vi "S4GUI.vi"() -> ()   [LabVIEW 2018] (continued)
            n2911 = call-dynamic "Write Temperature.vi"("error in (no error)"=w7074, "Temperature"="Target Temp 4", "Interface in"=w7075) -> ("error out"=w7070:errorcluster, "Interface out"=w7073:refnum<class "Interface.lvclass">)  [unwired: 7 in]
            n2912 = call-dynamic "Write Interface.vi"("error in (no error)"=w7070, "Interface.lvclass"=w7073, "Channel in"=w7072) -> ("error out"=w7069:errorcluster, "Channel out"=w7071:refnum<class "Channel.lvclass">)  [unwired: 7 in]
            n2913 = call-dynamic "Read State Machine.vi"("error in (no error)"=w7069, "Device in"=w7071) -> ("error out"=w7092:errorcluster, "State Machine.lvclass"=w7093:refnum<class "State Machine.lvclass">, "Device out"=w7089:refnum<class "Channel.lvclass">)  [unwired: 7 in]
            n2914 = call "Next State.vi"("error in (no error)"=w7092, "New_State"=u32 35, "State Machine in"=w7093) -> ("error out"=w7087:errorcluster, "State Machine out"=w7090:refnum<class "State Machine.lvclass">)  [unwired: 7 in]
            n2915 = call-dynamic "Write State Machine.vi"("error in (no error)"=w7087, "State Machine.lvclass"=w7090, "Device in"=w7089) -> ("error out"=w7083:errorcluster, "Device out"=w7082:refnum<class "Channel.lvclass">)  [unwired: 7 in]
            n2916 = call-dynamic "Write Channel.vi"("error in (no error)"=w7083, "Channel.lvclass"=w7082, "Acquisition in"=w7088) -> ("error out"=w7084:errorcluster, "Acquisition out"=w7086:refnum<class "Acquisition.lvclass">)  [unwired: 7 in]
            n2917 = call-dynamic "Write AcquisitionD.vi"("error in (no error)"=w7084, "Acquisition.lvclass"=w7086, "S4ACS_GUI in"=w7085) -> ("error out"=w7079:errorcluster, "S4ACS_GUI out"=w7078:refnum<class "S4GUI.lvclass">)  [unwired: 7 in]
          }
        }
      }
      event "Avança Estado": Value Change {
        n2918 = event-data() -> ()  [unwired: 1 in, 4 out]
        n2919 = call-dynamic "Read Sync Box.lvclass.vi"("error in (no error)"=w7104, "SPARC4_AC in"=w7105) -> ("error out"=w7117:errorcluster, "Sync Box.lvclass"=w7118:refnum<class "Sync Box.lvclass">, "SPARC4_AC out"=w7109:refnum<class "S4GUI.lvclass">)  [unwired: 7 in]
        n2920 = call-dynamic "Read Trigger.lvclass.vi"("error in (no error)"=w7117, "Sync Box in"=w7118) -> ("error out"=w7115:errorcluster, "Trigger.lvclass"=w7116:refnum<class "Trigger.lvclass">, "Sync Box out"=w7112:refnum<class "Sync Box.lvclass">)  [unwired: 7 in]
        n2921 = call-dynamic "Read State Machine.vi"("error in (no error)"=w7115, "Device in"=w7116) -> ("error out"=w7101:errorcluster, "State Machine.lvclass"=w7102:refnum<class "State Machine.lvclass">, "Device out"=w7113:refnum<class "Trigger.lvclass">)  [unwired: 7 in]
        n2922 = call-dynamic "Read State.vi"("error in (no error)"=w7101, "State Machine in"=w7102) -> ("error out"=w7097:errorcluster, "State"=w7100:i32, "State Machine out"=w7098:refnum<class "State Machine.lvclass">)  [unwired: 7 in]
        n2923 = Increment(x=w7100) -> (x+1=w7099:i32)
        n2924 = call "Next State.vi"("error in (no error)"=w7097, "New_State"=w7099, "State Machine in"=w7098) -> ("error out"=w7111:errorcluster, "State Machine out"=w7114:refnum<class "State Machine.lvclass">)  [unwired: 7 in]
        n2925 = call-dynamic "Write State Machine.vi"("error in (no error)"=w7111, "State Machine.lvclass"=w7114, "Device in"=w7113) -> ("error out"=w7107:errorcluster, "Device out"=w7106:refnum<class "Trigger.lvclass">)  [unwired: 7 in]
        n2926 = call-dynamic "Write Trigger.lvclass.vi"("error in (no error)"=w7107, "Trigger.lvclass"=w7106, "Sync Box in"=w7112) -> ("error out"=w7108:errorcluster, "Sync Box out"=w7110:refnum<class "Sync Box.lvclass">)  [unwired: 7 in]
        n2927 = call-dynamic "Write Sync Box.lvclass.vi"("error in (no error)"=w7108, "Sync Box.lvclass"=w7110, "SPARC4_AC in"=w7109) -> ("error out"=w7103:errorcluster, "SPARC4_AC out"=w7096:refnum<class "S4GUI.lvclass">)  [unwired: 7 in]
      }
      event "DelayA": Value Change {
        n2928 = event-data() -> ("NewVal"=w7120:string)  [unwired: 1 in, 3 out]
        n2929 = call-dynamic "Read Sync Box.lvclass.vi"("error in (no error)"=w7124, "SPARC4_AC in"=w7125) -> ("error out"=w7132:errorcluster, "Sync Box.lvclass"=w7133:refnum<class "Sync Box.lvclass">, "SPARC4_AC out"=w7129:refnum<class "S4GUI.lvclass">)  [unwired: 7 in]
        n2930 = call-dynamic "Read Trigger.lvclass.vi"("error in (no error)"=w7132, "Sync Box in"=w7133) -> ("error out"=w7121:errorcluster, "Trigger.lvclass"=w7122:refnum<class "Trigger.lvclass">, "Sync Box out"=w7131:refnum<class "Sync Box.lvclass">)  [unwired: 7 in]
        n2931 = call-dynamic "Write DelayA.vi"("error in (no error)"=w7121, "DelayA"=w7120, "Trigger in"=w7122) -> ("error out"=w7127:errorcluster, "Trigger out"=w7126:refnum<class "Trigger.lvclass">)  [unwired: 7 in]
        n2932 = call-dynamic "Write Trigger.lvclass.vi"("error in (no error)"=w7127, "Trigger.lvclass"=w7126, "Sync Box in"=w7131) -> ("error out"=w7128:errorcluster, "Sync Box out"=w7130:refnum<class "Sync Box.lvclass">)  [unwired: 7 in]
        n2933 = call-dynamic "Write Sync Box.lvclass.vi"("error in (no error)"=w7128, "Sync Box.lvclass"=w7130, "SPARC4_AC in"=w7129) -> ("error out"=w7123:errorcluster, "SPARC4_AC out"=w7119:refnum<class "S4GUI.lvclass">)  [unwired: 7 in]
      }
      event "DelayB": Value Change {
        n2934 = event-data() -> ("NewVal"=w7135:string)  [unwired: 1 in, 3 out]
        n2935 = call-dynamic "Read Sync Box.lvclass.vi"("error in (no error)"=w7139, "SPARC4_AC in"=w7140) -> ("error out"=w7147:errorcluster, "Sync Box.lvclass"=w7148:refnum<class "Sync Box.lvclass">, "SPARC4_AC out"=w7144:refnum<class "S4GUI.lvclass">)  [unwired: 7 in]
        n2936 = call-dynamic "Read Trigger.lvclass.vi"("error in (no error)"=w7147, "Sync Box in"=w7148) -> ("error out"=w7136:errorcluster, "Trigger.lvclass"=w7137:refnum<class "Trigger.lvclass">, "Sync Box out"=w7146:refnum<class "Sync Box.lvclass">)  [unwired: 7 in]
        n2937 = call-dynamic "Write DelayB.vi"("error in (no error)"=w7136, "DelayB"=w7135, "Trigger in"=w7137) -> ("error out"=w7142:errorcluster, "Trigger out"=w7141:refnum<class "Trigger.lvclass">)  [unwired: 7 in]
        n2938 = call-dynamic "Write Trigger.lvclass.vi"("error in (no error)"=w7142, "Trigger.lvclass"=w7141, "Sync Box in"=w7146) -> ("error out"=w7143:errorcluster, "Sync Box out"=w7145:refnum<class "Sync Box.lvclass">)  [unwired: 7 in]
        n2939 = call-dynamic "Write Sync Box.lvclass.vi"("error in (no error)"=w7143, "Sync Box.lvclass"=w7145, "SPARC4_AC in"=w7144) -> ("error out"=w7138:errorcluster, "SPARC4_AC out"=w7134:refnum<class "S4GUI.lvclass">)  [unwired: 7 in]
      }
      event "DelayC": Value Change {
        n2940 = event-data() -> ("NewVal"=w7150:string)  [unwired: 1 in, 3 out]
        n2941 = call-dynamic "Read Sync Box.lvclass.vi"("error in (no error)"=w7154, "SPARC4_AC in"=w7155) -> ("error out"=w7162:errorcluster, "Sync Box.lvclass"=w7163:refnum<class "Sync Box.lvclass">, "SPARC4_AC out"=w7159:refnum<class "S4GUI.lvclass">)  [unwired: 7 in]
        n2942 = call-dynamic "Read Trigger.lvclass.vi"("error in (no error)"=w7162, "Sync Box in"=w7163) -> ("error out"=w7151:errorcluster, "Trigger.lvclass"=w7152:refnum<class "Trigger.lvclass">, "Sync Box out"=w7161:refnum<class "Sync Box.lvclass">)  [unwired: 7 in]
        n2943 = call-dynamic "Write DelayC.vi"("error in (no error)"=w7151, "DelayC"=w7150, "Trigger in"=w7152) -> ("error out"=w7157:errorcluster, "Trigger out"=w7156:refnum<class "Trigger.lvclass">)  [unwired: 7 in]
        n2944 = call-dynamic "Write Trigger.lvclass.vi"("error in (no error)"=w7157, "Trigger.lvclass"=w7156, "Sync Box in"=w7161) -> ("error out"=w7158:errorcluster, "Sync Box out"=w7160:refnum<class "Sync Box.lvclass">)  [unwired: 7 in]
        n2945 = call-dynamic "Write Sync Box.lvclass.vi"("error in (no error)"=w7158, "Sync Box.lvclass"=w7160, "SPARC4_AC in"=w7159) -> ("error out"=w7153:errorcluster, "SPARC4_AC out"=w7149:refnum<class "S4GUI.lvclass">)  [unwired: 7 in]
      }
      event "DelayD": Value Change {
        n2946 = event-data() -> ("NewVal"=w7165:string)  [unwired: 1 in, 3 out]
        n2947 = call-dynamic "Read Sync Box.lvclass.vi"("error in (no error)"=w7169, "SPARC4_AC in"=w7170) -> ("error out"=w7177:errorcluster, "Sync Box.lvclass"=w7178:refnum<class "Sync Box.lvclass">, "SPARC4_AC out"=w7174:refnum<class "S4GUI.lvclass">)  [unwired: 7 in]
        n2948 = call-dynamic "Read Trigger.lvclass.vi"("error in (no error)"=w7177, "Sync Box in"=w7178) -> ("error out"=w7166:errorcluster, "Trigger.lvclass"=w7167:refnum<class "Trigger.lvclass">, "Sync Box out"=w7176:refnum<class "Sync Box.lvclass">)  [unwired: 7 in]
        n2949 = call-dynamic "Write DelayD.vi"("error in (no error)"=w7166, "DelayD"=w7165, "Trigger in"=w7167) -> ("error out"=w7172:errorcluster, "Trigger out"=w7171:refnum<class "Trigger.lvclass">)  [unwired: 7 in]
        n2950 = call-dynamic "Write Trigger.lvclass.vi"("error in (no error)"=w7172, "Trigger.lvclass"=w7171, "Sync Box in"=w7176) -> ("error out"=w7173:errorcluster, "Sync Box out"=w7175:refnum<class "Sync Box.lvclass">)  [unwired: 7 in]
        n2951 = call-dynamic "Write Sync Box.lvclass.vi"("error in (no error)"=w7173, "Sync Box.lvclass"=w7175, "SPARC4_AC in"=w7174) -> ("error out"=w7168:errorcluster, "SPARC4_AC out"=w7164:refnum<class "S4GUI.lvclass">)  [unwired: 7 in]
      }
      event "WidthA": Value Change {
        n2952 = event-data() -> ("NewVal"=w7180:string)  [unwired: 1 in, 3 out]
        n2953 = call-dynamic "Read Sync Box.lvclass.vi"("error in (no error)"=w7184, "SPARC4_AC in"=w7185) -> ("error out"=w7192:errorcluster, "Sync Box.lvclass"=w7193:refnum<class "Sync Box.lvclass">, "SPARC4_AC out"=w7189:refnum<class "S4GUI.lvclass">)  [unwired: 7 in]
        n2954 = call-dynamic "Read Trigger.lvclass.vi"("error in (no error)"=w7192, "Sync Box in"=w7193) -> ("error out"=w7181:errorcluster, "Trigger.lvclass"=w7182:refnum<class "Trigger.lvclass">, "Sync Box out"=w7191:refnum<class "Sync Box.lvclass">)  [unwired: 7 in]
        n2955 = call-dynamic "Write WidthA.vi"("error in (no error)"=w7181, "WidthA"=w7180, "Trigger in"=w7182) -> ("error out"=w7187:errorcluster, "Trigger out"=w7186:refnum<class "Trigger.lvclass">)  [unwired: 7 in]
        n2956 = call-dynamic "Write Trigger.lvclass.vi"("error in (no error)"=w7187, "Trigger.lvclass"=w7186, "Sync Box in"=w7191) -> ("error out"=w7188:errorcluster, "Sync Box out"=w7190:refnum<class "Sync Box.lvclass">)  [unwired: 7 in]
        n2957 = call-dynamic "Write Sync Box.lvclass.vi"("error in (no error)"=w7188, "Sync Box.lvclass"=w7190, "SPARC4_AC in"=w7189) -> ("error out"=w7183:errorcluster, "SPARC4_AC out"=w7179:refnum<class "S4GUI.lvclass">)  [unwired: 7 in]
      }
      event "WidthB": Value Change {
        n2958 = event-data() -> ("NewVal"=w7195:string)  [unwired: 1 in, 3 out]
        n2959 = call-dynamic "Read Sync Box.lvclass.vi"("error in (no error)"=w7199, "SPARC4_AC in"=w7200) -> ("error out"=w7207:errorcluster, "Sync Box.lvclass"=w7208:refnum<class "Sync Box.lvclass">, "SPARC4_AC out"=w7204:refnum<class "S4GUI.lvclass">)  [unwired: 7 in]
        n2960 = call-dynamic "Read Trigger.lvclass.vi"("error in (no error)"=w7207, "Sync Box in"=w7208) -> ("error out"=w7196:errorcluster, "Trigger.lvclass"=w7197:refnum<class "Trigger.lvclass">, "Sync Box out"=w7206:refnum<class "Sync Box.lvclass">)  [unwired: 7 in]
        n2961 = call-dynamic "Write WidthB.vi"("error in (no error)"=w7196, "WidthB"=w7195, "Trigger in"=w7197) -> ("error out"=w7202:errorcluster, "Trigger out"=w7201:refnum<class "Trigger.lvclass">)  [unwired: 7 in]
        n2962 = call-dynamic "Write Trigger.lvclass.vi"("error in (no error)"=w7202, "Trigger.lvclass"=w7201, "Sync Box in"=w7206) -> ("error out"=w7203:errorcluster, "Sync Box out"=w7205:refnum<class "Sync Box.lvclass">)  [unwired: 7 in]
        n2963 = call-dynamic "Write Sync Box.lvclass.vi"("error in (no error)"=w7203, "Sync Box.lvclass"=w7205, "SPARC4_AC in"=w7204) -> ("error out"=w7198:errorcluster, "SPARC4_AC out"=w7194:refnum<class "S4GUI.lvclass">)  [unwired: 7 in]
      }
      event "WidthC": Value Change {
        n2964 = event-data() -> ("NewVal"=w7210:string)  [unwired: 1 in, 3 out]
        n2965 = call-dynamic "Read Sync Box.lvclass.vi"("error in (no error)"=w7214, "SPARC4_AC in"=w7215) -> ("error out"=w7222:errorcluster, "Sync Box.lvclass"=w7223:refnum<class "Sync Box.lvclass">, "SPARC4_AC out"=w7219:refnum<class "S4GUI.lvclass">)  [unwired: 7 in]
        n2966 = call-dynamic "Read Trigger.lvclass.vi"("error in (no error)"=w7222, "Sync Box in"=w7223) -> ("error out"=w7211:errorcluster, "Trigger.lvclass"=w7212:refnum<class "Trigger.lvclass">, "Sync Box out"=w7221:refnum<class "Sync Box.lvclass">)  [unwired: 7 in]
        n2967 = call-dynamic "Write WidthC.vi"("error in (no error)"=w7211, "WidthC"=w7210, "Trigger in"=w7212) -> ("error out"=w7217:errorcluster, "Trigger out"=w7216:refnum<class "Trigger.lvclass">)  [unwired: 7 in]
        n2968 = call-dynamic "Write Trigger.lvclass.vi"("error in (no error)"=w7217, "Trigger.lvclass"=w7216, "Sync Box in"=w7221) -> ("error out"=w7218:errorcluster, "Sync Box out"=w7220:refnum<class "Sync Box.lvclass">)  [unwired: 7 in]
        n2969 = call-dynamic "Write Sync Box.lvclass.vi"("error in (no error)"=w7218, "Sync Box.lvclass"=w7220, "SPARC4_AC in"=w7219) -> ("error out"=w7213:errorcluster, "SPARC4_AC out"=w7209:refnum<class "S4GUI.lvclass">)  [unwired: 7 in]
      }
      event "WidthD": Value Change {
        n2970 = event-data() -> ("NewVal"=w7225:string)  [unwired: 1 in, 3 out]
        n2971 = call-dynamic "Read Sync Box.lvclass.vi"("error in (no error)"=w7229, "SPARC4_AC in"=w7230) -> ("error out"=w7237:errorcluster, "Sync Box.lvclass"=w7238:refnum<class "Sync Box.lvclass">, "SPARC4_AC out"=w7234:refnum<class "S4GUI.lvclass">)  [unwired: 7 in]
        n2972 = call-dynamic "Read Trigger.lvclass.vi"("error in (no error)"=w7237, "Sync Box in"=w7238) -> ("error out"=w7226:errorcluster, "Trigger.lvclass"=w7227:refnum<class "Trigger.lvclass">, "Sync Box out"=w7236:refnum<class "Sync Box.lvclass">)  [unwired: 7 in]
        n2973 = call-dynamic "Write WidthD.vi"("error in (no error)"=w7226, "WidthD"=w7225, "Trigger in"=w7227) -> ("error out"=w7232:errorcluster, "Trigger out"=w7231:refnum<class "Trigger.lvclass">)  [unwired: 7 in]
        n2974 = call-dynamic "Write Trigger.lvclass.vi"("error in (no error)"=w7232, "Trigger.lvclass"=w7231, "Sync Box in"=w7236) -> ("error out"=w7233:errorcluster, "Sync Box out"=w7235:refnum<class "Sync Box.lvclass">)  [unwired: 7 in]
        n2975 = call-dynamic "Write Sync Box.lvclass.vi"("error in (no error)"=w7233, "Sync Box.lvclass"=w7235, "SPARC4_AC in"=w7234) -> ("error out"=w7228:errorcluster, "SPARC4_AC out"=w7224:refnum<class "S4GUI.lvclass">)  [unwired: 7 in]
      }
      event "WPROT_set": Value Change {
        # "Espera até 10 x 1s = 10s\npara condition de WPROT\n ir para READY"
        n2976 = event-data() -> ()  [unwired: 1 in, 4 out]
        n2977 = call "Read Instrument.lvclass.vi"("error in (no error)"=w7260, "S4ACS_GUI in"=w7261) -> ("error out"=w7258:errorcluster, "Instrument.lvclass"=w7259:refnum<class "Instrument.lvclass">, "S4ACS_GUI out"=w7247:refnum<class "S4GUI.lvclass">)  [unwired: 7 in]
        n2978 = call "Read WPROT.vi"("error in (no error)"=w7258, "Instrument in"=w7259) -> ("error out"=w7254:errorcluster, "Opt_Selector.lvclass"=w7257:refnum<class "Opt_Selector.lvclass">, "Instrument out"=w7250:refnum<class "Instrument.lvclass">)  [unwired: 7 in]
        n2979 = call-dynamic "Read State Machine.vi"("error in (no error)"=w7254, "Device in"=w7257) -> ("error out"=w7253:errorcluster, "State Machine.lvclass"=w7256:refnum<class "State Machine.lvclass">, "Device out"=w7252:refnum<class "Opt_Selector.lvclass">)  [unwired: 7 in]
        n2980 = call "Next State.vi"("error in (no error)"=w7253, "New_State"=1, "State Machine in"=w7256) -> ("error out"=w7241:errorcluster, "State Machine out"=w7243:refnum<class "State Machine.lvclass">)  [unwired: 7 in]
        n2981 = call-dynamic "Write Timer.vi"("error in (no error)"=w7241, "Timer"=u32 10, "State Machine in"=w7243) -> ("error out"=w7240:errorcluster, "State Machine out"=w7242:refnum<class "State Machine.lvclass">)  [unwired: 7 in]
        n2982 = call-dynamic "Write State Machine.vi"("error in (no error)"=w7240, "State Machine.lvclass"=w7242, "Device in"=w7252) -> ("error out"=w7249:errorcluster, "Device out"=w7251:refnum<class "Opt_Selector.lvclass">)  [unwired: 7 in]
        n2983 = call "Write WPROT.vi"("error in (no error)"=w7249, "Opt_Selector.lvclass"=w7251, "Instrument in"=w7250) -> ("error out"=w7246:errorcluster, "Instrument out"=w7248:refnum<class "Instrument.lvclass">)  [unwired: 7 in]
        n2984 = call "Write Instrument.lvclass.vi"("error in (no error)"=w7246, "Instrument.lvclass"=w7248, "S4ACS_GUI in"=w7247) -> ("error out"=w7245:errorcluster, "S4ACS_GUI out"=w7244:refnum<class "S4GUI.lvclass">)  [unwired: 7 in]
      }
      event "TARGET NAME WPROT": Value Change {
        n2985 = event-data() -> ()  [unwired: 1 in, 1 out]
        n2986 = property on="TARGET NAME WPROT" class="Enum (strict)"() -> ("RingText.Text"=w7288:string)  [unwired: 2 in, 2 out]
        n2987 = call "Read Instrument.lvclass.vi"("error in (no error)"=w7289, "S4ACS_GUI in"=w7290) -> ("error out"=w7297:errorcluster, "Instrument.lvclass"=w7298:refnum<class "Instrument.lvclass">, "S4ACS_GUI out"=w7292:refnum<class "S4GUI.lvclass">)  [unwired: 7 in]
        n2988 = Build Array(-1.0 ("element"), 0.0 ("element"), 22.5 ("element"), 45.0 ("element"), 67.5 ("element"), 90.0 ("element"), 112.5 ("element"), 135.0 ("element"), 157.5 ("element"), 180.0 ("element"), 202.5 ("element"), 225.0 ("element"), 247.5 ("element"), 270.0 ("element"), 292.5 ("element"), 315.0 ("element"), 337.5 ("element")) -> (w7280:dbl[])
        n2989 = call "Read WPROT.vi"("error in (no error)"=w7297, "Instrument in"=w7298) -> ("error out"=w7295:errorcluster, "Opt_Selector.lvclass"=w7296:refnum<class "Opt_Selector.lvclass">, "Instrument out"=w7294:refnum<class "Instrument.lvclass">)  [unwired: 7 in]
        n2990 = call "Write target name.vi"("error in (no error)"=w7295, "target name"=w7288, "Optics in"=w7296) -> ("error out"=w7276:errorcluster, "Optics out"=w7277:refnum<class "Opt_Selector.lvclass">)  [unwired: 7 in]
        n2991 = Index Array(array=w7280, index="TARGET NAME WPROT") -> (element=w7278:dbl)
        n2992 = call "Write target.vi"("error in (no error)"=w7276, "target"=w7278, "Optics in"=w7277) -> ("error out"=w7275:errorcluster, "Optics out"=w7274:refnum<class "Opt_Selector.lvclass">)  [unwired: 7 in]
        n2993 = call "Write WPROT.vi"("error in (no error)"=w7275, "Opt_Selector.lvclass"=w7274, "Instrument in"=w7294) -> ("error out"=w7291:errorcluster, "Instrument out"=w7293:refnum<class "Instrument.lvclass">)  [unwired: 7 in]
        n2994 = call "Write Instrument.lvclass.vi"("error in (no error)"=w7291, "Instrument.lvclass"=w7293, "S4ACS_GUI in"=w7292) -> ("error out"=w7287:errorcluster, "S4ACS_GUI out"=w7262:refnum<class "S4GUI.lvclass">)  [unwired: 7 in]
      }
      event "TARGET NAME WPSEL": Value Change {
        n2995 = event-data() -> ()  [unwired: 1 in, 1 out]
        n2996 = property on="TARGET NAME WPSEL" class="Enum (strict)"() -> ("RingText.Text"=w7300:string)  [unwired: 2 in, 2 out]
        n2997 = call "Read Instrument.lvclass.vi"("error in (no error)"=w7313, "S4ACS_GUI in"=w7314) -> ("error out"=w7321:errorcluster, "Instrument.lvclass"=w7322:refnum<class "Instrument.lvclass">, "S4ACS_GUI out"=w7316:refnum<class "S4GUI.lvclass">)  [unwired: 7 in]
        n2998 = Build Array(-1.0 ("element"), 80.0 ("element"), 0.0 ("element"), 160.0 ("element")) -> (w7307:dbl[])
        n2999 = call "Read WPSEL.vi"("error in (no error)"=w7321, "Instrument in"=w7322) -> ("error out"=w7319:errorcluster, "Opt_Selector.lvclass"=w7320:refnum<class "Opt_Selector.lvclass">, "Instrument out"=w7318:refnum<class "Instrument.lvclass">)  [unwired: 7 in]
        n3000 = call "Write target name.vi"("error in (no error)"=w7319, "target name"=w7300, "Optics in"=w7320) -> ("error out"=w7304:errorcluster, "Optics out"=w7305:refnum<class "Opt_Selector.lvclass">)  [unwired: 7 in]
        n3001 = Index Array(array=w7307, index="TARGET NAME WPSEL") -> (element=w7306:dbl)
        n3002 = call "Write target.vi"("error in (no error)"=w7304, "target"=w7306, "Optics in"=w7305) -> ("error out"=w7303:errorcluster, "Optics out"=w7302:refnum<class "Opt_Selector.lvclass">)  [unwired: 7 in]
        n3003 = call "Write WPSEL.vi"("error in (no error)"=w7303, "Opt_Selector.lvclass"=w7302, "Instrument in"=w7318) -> ("error out"=w7315:errorcluster, "Instrument out"=w7317:refnum<class "Instrument.lvclass">)  [unwired: 7 in]
        n3004 = call "Write Instrument.lvclass.vi"("error in (no error)"=w7315, "Instrument.lvclass"=w7317, "S4ACS_GUI in"=w7316) -> ("error out"=w7312:errorcluster, "S4ACS_GUI out"=w7299:refnum<class "S4GUI.lvclass">)  [unwired: 7 in]
      }
      event "Lambda Selector": Value Change {
        n3005 = event-data() -> ("NewVal"=w7324:u16)  [unwired: 1 in, 1 out]
        n3006 = property on="Lambda Selector" class="Ring (strict)"() -> ("RingText.Text"=w7330:string)  [unwired: 2 in, 2 out]
        n3007 = call "Read Instrument.lvclass.vi"("error in (no error)"=w7355, "S4ACS_GUI in"=w7356) -> ("error out"=w7357:errorcluster, "Instrument.lvclass"=w7332:refnum<class "Instrument.lvclass">, "S4ACS_GUI out"=w7329:refnum<class "S4GUI.lvclass">)  [unwired: 7 in]
        n3008 = Build Array(80.0 ("element"), 0.0 ("element"), 160.0 ("element")) -> (w7350:dbl[])
        n3009 = call "Read WPSEL.vi"("error in (no error)"=w7357, "Instrument in"=w7332) -> ("error out"=w7339:errorcluster, "Opt_Selector.lvclass"=w7338:refnum<class "Opt_Selector.lvclass">, "Instrument out"=w7331:refnum<class "Instrument.lvclass">)  [unwired: 7 in]
        n3010 = Index Array(array=w7350, index=w7324) -> (element=w7349:dbl)
        n3011 = call "Write target.vi"("error in (no error)"=w7339, "target"=w7349, "Optics in"=w7338) -> ("error out"=w7336:errorcluster, "Optics out"=w7337:refnum<class "Opt_Selector.lvclass">)  [unwired: 7 in]
        n3012 = case shown="\"Lambda/2\"" w7330 {
          selector: w7330 -> [w7360 _ _]
          tunnel: [w7360 "ON" "ON"] -> w7341
          tunnel: [0.0 ("element") 30.0 ("element") 30.0 ("element")] -> w7340
          tunnel: [w7360 "L/2" "L/4"] -> w7333
          frame "OFF", Default {
            n3013 = property on="Calibrator Selector" class="Ring (strict)"("DisabledEnum"=T7."Disabled and Grayed Out" ("Disabled")) -> ()  [unwired: 2 in, 2 out]
          }
          frame "Lambda/2" {
            n3014 = property on="Calibrator Selector" class="Ring (strict)"("DisabledEnum"=T7."Enabled" ("Disabled")) -> ()  [unwired: 2 in, 2 out]
          }
          frame "Lambda/4" {
            n3015 = property on="Calibrator Selector" class="Ring (strict)"("DisabledEnum"=T7."Enabled" ("Disabled")) -> ()  [unwired: 2 in, 2 out]
          }
        }
        n3016 = call "Write target name.vi"("error in (no error)"=w7336, "target name"=w7333, "Optics in"=w7337) -> ("error out"=w7335:errorcluster, "Optics out"=w7334:refnum<class "Opt_Selector.lvclass">)  [unwired: 7 in]
        n3017 = call "Write WPSEL.vi"("error in (no error)"=w7335, "Opt_Selector.lvclass"=w7334, "Instrument in"=w7331) -> ("error out"=w7326:errorcluster, "Instrument out"=w7325:refnum<class "Instrument.lvclass">)  [unwired: 7 in]
        n3018 = call "Read ASEL.vi"("error in (no error)"=w7326, "Instrument in"=w7325) -> ("error out"=w7346:errorcluster, "Opt_Selector.lvclass"=w7344:refnum<class "Opt_Selector.lvclass">, "Instrument out"=w7328:refnum<class "Instrument.lvclass">)  [unwired: 7 in]
        n3019 = call "Write target name.vi"("error in (no error)"=w7346, "target name"=w7341, "Optics in"=w7344) -> ("error out"=w7347:errorcluster, "Optics out"=w7343:refnum<class "Opt_Selector.lvclass">)  [unwired: 7 in]
        n3020 = call "Write target.vi"("error in (no error)"=w7347, "target"=w7340, "Optics in"=w7343) -> ("error out"=w7348:errorcluster, "Optics out"=w7342:refnum<class "Opt_Selector.lvclass">)  [unwired: 7 in]
        n3021 = call "Write ASEL.vi"("error in (no error)"=w7348, "Opt_Selector.lvclass"=w7342, "Instrument in"=w7328) -> ("error out"=w7345:errorcluster, "Instrument out"=w7327:refnum<class "Instrument.lvclass">)  [unwired: 7 in]
        n3022 = call "Write Instrument.lvclass.vi"("error in (no error)"=w7345, "Instrument.lvclass"=w7327, "S4ACS_GUI in"=w7329) -> ("error out"=w7354:errorcluster, "S4ACS_GUI out"=w7323:refnum<class "S4GUI.lvclass">)  [unwired: 7 in]
      }
      event "Calibrator Selector": Value Change {
        n3023 = event-data() -> ()  [unwired: 1 in, 6 out]
        n3024 = call "Read Instrument.lvclass.vi"("error in (no error)"=w7389, "S4ACS_GUI in"=w7390) -> ("error out"=w7393:errorcluster, "Instrument.lvclass"=w7394:refnum<class "Instrument.lvclass">, "S4ACS_GUI out"=w7391:refnum<class "S4GUI.lvclass">)  [unwired: 7 in]
        n3025 = property on="Calibrator Selector" class="Ring (strict)"() -> ("RingText.Text"=w7375:string)  [unwired: 2 in, 2 out]
        n3026 = Build Array(0.0 ("element"), 72.0 ("element"), 144.0 ("element"), 216.0 ("element"), 288.0 ("element")) -> (w7384:dbl[])
        n3027 = call "Read CALW.vi"("error in (no error)"=w7393, "Instrument in"=w7394) -> ("error out"=w7382:errorcluster, "Opt_Selector.lvclass"=w7381:refnum<class "Opt_Selector.lvclass">, "Instrument out"=w7392:refnum<class "Instrument.lvclass">)  [unwired: 7 in]
        n3028 = Index Array(array=w7384, index="Calibrator Selector") -> (element=w7383:dbl)
        n3029 = call "Write target.vi"("error in (no error)"=w7382, "target"=w7383, "Optics in"=w7381) -> ("error out"=w7379:errorcluster, "Optics out"=w7380:refnum<class "Opt_Selector.lvclass">)  [unwired: 7 in]
        n3030 = case shown="\"POLARIZER\"" w7375 {
          selector: w7375 -> [_ w7396 w7397 w7398 w7399]
          tunnel: ["OFF" w7396 w7397 w7398 w7399] -> w7376
          frame "OFF", Default {
          }
          frame "POLARIZER" {
          }
          frame "DEPOLARIZER" {
          }
          frame "PINHOLE" {
          }
          frame "SHUTTER" {
          }
        }
        n3031 = call "Write target name.vi"("error in (no error)"=w7379, "target name"=w7376, "Optics in"=w7380) -> ("error out"=w7378:errorcluster, "Optics out"=w7377:refnum<class "Opt_Selector.lvclass">)  [unwired: 7 in]
        n3032 = call "Write CALW.vi"("error in (no error)"=w7378, "Opt_Selector.lvclass"=w7377, "Instrument in"=w7392) -> ("error out"=w7372:errorcluster, "Instrument out"=w7373:refnum<class "Instrument.lvclass">)  [unwired: 7 in]
        n3033 = call "Write Instrument.lvclass.vi"("error in (no error)"=w7372, "Instrument.lvclass"=w7373, "S4ACS_GUI in"=w7391) -> ("error out"=w7388:errorcluster, "S4ACS_GUI out"=w7371:refnum<class "S4GUI.lvclass">)  [unwired: 7 in]
      }
      event "TARGET NAME CALW": Value Change {
        # "aqui também"
        # "aqui também"
        # "OV20230426: Montagem do CALW\nestá POL e DEPOL invertidos"
        n3034 = event-data() -> ()  [unwired: 1 in, 6 out]
        n3035 = property on="TARGET NAME CALW" class="Enum (strict)"() -> ("RingText.Text"=w7401:string)  [unwired: 2 in, 2 out]
        n3036 = case shown="Default" w7401 {
          selector: w7401 -> [_ _ w7429]
          tunnel: ["DEPOLARIZER" "POLARIZER" w7429] -> w7400
          frame "POLARIZER" {
          }
          frame "DEPOLARIZER" {
          }
          frame Default {
          }
        }
        n3037 = call "Read Instrument.lvclass.vi"("error in (no error)"=w7417, "S4ACS_GUI in"=w7418) -> ("error out"=w7425:errorcluster, "Instrument.lvclass"=w7426:refnum<class "Instrument.lvclass">, "S4ACS_GUI out"=w7420:refnum<class "S4GUI.lvclass">)  [unwired: 7 in]
        n3038 = Build Array(-1.0 ("element"), 0.0 ("element"), 288.0 ("element"), 144.0 ("element"), 216.0 ("element"), 72.0 ("element")) -> (w7411:dbl[])
        n3039 = call "Read CALW.vi"("error in (no error)"=w7425, "Instrument in"=w7426) -> ("error out"=w7423:errorcluster, "Opt_Selector.lvclass"=w7424:refnum<class "Opt_Selector.lvclass">, "Instrument out"=w7422:refnum<class "Instrument.lvclass">)  [unwired: 7 in]
        n3040 = call "Write target name.vi"("error in (no error)"=w7423, "target name"=w7400, "Optics in"=w7424) -> ("error out"=w7408:errorcluster, "Optics out"=w7409:refnum<class "Opt_Selector.lvclass">)  [unwired: 7 in]
        n3041 = Index Array(array=w7411, index="TARGET NAME CALW") -> (element=w7410:dbl)
        n3042 = call "Write target.vi"("error in (no error)"=w7408, "target"=w7410, "Optics in"=w7409) -> ("error out"=w7407:errorcluster, "Optics out"=w7406:refnum<class "Opt_Selector.lvclass">)  [unwired: 7 in]
        n3043 = call "Write CALW.vi"("error in (no error)"=w7407, "Opt_Selector.lvclass"=w7406, "Instrument in"=w7422) -> ("error out"=w7419:errorcluster, "Instrument out"=w7421:refnum<class "Instrument.lvclass">)  [unwired: 7 in]
        n3044 = call "Write Instrument.lvclass.vi"("error in (no error)"=w7419, "Instrument.lvclass"=w7421, "S4ACS_GUI in"=w7420) -> ("error out"=w7416:errorcluster, "S4ACS_GUI out"=w7402:refnum<class "S4GUI.lvclass">)  [unwired: 7 in]
      }
      event "TARGET NAME ASEL": Value Change {
        n3045 = event-data() -> ()  [unwired: 1 in, 6 out]
        n3046 = property on="TARGET NAME ASEL" class="Enum (strict)"() -> ("RingText.Text"=w7432:string)  [unwired: 2 in, 2 out]
        n3047 = call "Read Instrument.lvclass.vi"("error in (no error)"=w7443, "S4ACS_GUI in"=w7444) -> ("error out"=w7451:errorcluster, "Instrument.lvclass"=w7452:refnum<class "Instrument.lvclass">, "S4ACS_GUI out"=w7446:refnum<class "S4GUI.lvclass">)  [unwired: 7 in]
        n3048 = Build Array(-1.0 ("element"), 0.0 ("element"), 30.0 ("element")) -> (w7438:dbl[])
        n3049 = call "Read ASEL.vi"("error in (no error)"=w7451, "Instrument in"=w7452) -> ("error out"=w7449:errorcluster, "Opt_Selector.lvclass"=w7450:refnum<class "Opt_Selector.lvclass">, "Instrument out"=w7448:refnum<class "Instrument.lvclass">)  [unwired: 7 in]
        n3050 = call "Write target name.vi"("error in (no error)"=w7449, "target name"=w7432, "Optics in"=w7450) -> ("error out"=w7435:errorcluster, "Optics out"=w7436:refnum<class "Opt_Selector.lvclass">)  [unwired: 7 in]
        n3051 = Index Array(array=w7438, index="TARGET NAME ASEL") -> (element=w7437:dbl)
        n3052 = call "Write target.vi"("error in (no error)"=w7435, "target"=w7437, "Optics in"=w7436) -> ("error out"=w7434:errorcluster, "Optics out"=w7433:refnum<class "Opt_Selector.lvclass">)  [unwired: 7 in]
        n3053 = call "Write ASEL.vi"("error in (no error)"=w7434, "Opt_Selector.lvclass"=w7433, "Instrument in"=w7448) -> ("error out"=w7445:errorcluster, "Instrument out"=w7447:refnum<class "Instrument.lvclass">)  [unwired: 7 in]
        n3054 = call "Write Instrument.lvclass.vi"("error in (no error)"=w7445, "Instrument.lvclass"=w7447, "S4ACS_GUI in"=w7446) -> ("error out"=w7442:errorcluster, "S4ACS_GUI out"=w7430:refnum<class "S4GUI.lvclass">)  [unwired: 7 in]
      }
      event "WPROT_stop": Value Change {
        n3055 = event-data() -> ()  [unwired: 1 in, 4 out]
        n3056 = call "Read Instrument.lvclass.vi"("error in (no error)"=w7471, "S4ACS_GUI in"=w7472) -> ("error out"=w7469:errorcluster, "Instrument.lvclass"=w7470:refnum<class "Instrument.lvclass">, "S4ACS_GUI out"=w7456:refnum<class "S4GUI.lvclass">)  [unwired: 7 in]
        n3057 = call "Read WPROT.vi"("error in (no error)"=w7469, "Instrument in"=w7470) -> ("error out"=w7465:errorcluster, "Opt_Selector.lvclass"=w7468:refnum<class "Opt_Selector.lvclass">, "Instrument out"=w7459:refnum<class "Instrument.lvclass">)  [unwired: 7 in]
        n3058 = call-dynamic "Read State Machine.vi"("error in (no error)"=w7465, "Device in"=w7468) -> ("error out"=w7464:errorcluster, "State Machine.lvclass"=w7467:refnum<class "State Machine.lvclass">, "Device out"=w7461:refnum<class "Opt_Selector.lvclass">)  [unwired: 7 in]
        n3059 = call "Next State.vi"("error in (no error)"=w7464, "New_State"=10, "State Machine in"=w7467) -> ("error out"=w7463:errorcluster, "State Machine out"=w7462:refnum<class "State Machine.lvclass">)  [unwired: 7 in]
        n3060 = call-dynamic "Write State Machine.vi"("error in (no error)"=w7463, "State Machine.lvclass"=w7462, "Device in"=w7461) -> ("error out"=w7458:errorcluster, "Device out"=w7460:refnum<class "Opt_Selector.lvclass">)  [unwired: 7 in]
        n3061 = call "Write WPROT.vi"("error in (no error)"=w7458, "Opt_Selector.lvclass"=w7460, "Instrument in"=w7459) -> ("error out"=w7455:errorcluster, "Instrument out"=w7457:refnum<class "Instrument.lvclass">)  [unwired: 7 in]
        n3062 = call "Write Instrument.lvclass.vi"("error in (no error)"=w7455, "Instrument.lvclass"=w7457, "S4ACS_GUI in"=w7456) -> ("error out"=w7454:errorcluster, "S4ACS_GUI out"=w7453:refnum<class "S4GUI.lvclass">)  [unwired: 7 in]
      }
      event "WPROT_init": Value Change {
        n3063 = event-data() -> ()  [unwired: 1 in, 4 out]
        n3064 = call "Read Instrument.lvclass.vi"("error in (no error)"=w7491, "S4ACS_GUI in"=w7492) -> ("error out"=w7489:errorcluster, "Instrument.lvclass"=w7490:refnum<class "Instrument.lvclass">, "S4ACS_GUI out"=w7476:refnum<class "S4GUI.lvclass">)  [unwired: 7 in]
        n3065 = call "Read WPROT.vi"("error in (no error)"=w7489, "Instrument in"=w7490) -> ("error out"=w7485:errorcluster, "Opt_Selector.lvclass"=w7488:refnum<class "Opt_Selector.lvclass">, "Instrument out"=w7479:refnum<class "Instrument.lvclass">)  [unwired: 7 in]
        n3066 = call-dynamic "Read State Machine.vi"("error in (no error)"=w7485, "Device in"=w7488) -> ("error out"=w7484:errorcluster, "State Machine.lvclass"=w7487:refnum<class "State Machine.lvclass">, "Device out"=w7481:refnum<class "Opt_Selector.lvclass">)  [unwired: 7 in]
        n3067 = call "Next State.vi"("error in (no error)"=w7484, "New_State"=30, "State Machine in"=w7487) -> ("error out"=w7483:errorcluster, "State Machine out"=w7482:refnum<class "State Machine.lvclass">)  [unwired: 7 in]
        n3068 = call-dynamic "Write State Machine.vi"("error in (no error)"=w7483, "State Machine.lvclass"=w7482, "Device in"=w7481) -> ("error out"=w7478:errorcluster, "Device out"=w7480:refnum<class "Opt_Selector.lvclass">)  [unwired: 7 in]
        n3069 = call "Write WPROT.vi"("error in (no error)"=w7478, "Opt_Selector.lvclass"=w7480, "Instrument in"=w7479) -> ("error out"=w7475:errorcluster, "Instrument out"=w7477:refnum<class "Instrument.lvclass">)  [unwired: 7 in]
        n3070 = call "Write Instrument.lvclass.vi"("error in (no error)"=w7475, "Instrument.lvclass"=w7477, "S4ACS_GUI in"=w7476) -> ("error out"=w7474:errorcluster, "S4ACS_GUI out"=w7473:refnum<class "S4GUI.lvclass">)  [unwired: 7 in]
      }
      event "WPSEL_target": Value Change {
        n3071 = event-data() -> ("NewVal"=w7502:dbl)  [unwired: 1 in, 3 out]
        n3072 = call "Read Instrument.lvclass.vi"("error in (no error)"=w7506, "S4ACS_GUI in"=w7507) -> ("error out"=w7504:errorcluster, "Instrument.lvclass"=w7505:refnum<class "Instrument.lvclass">, "S4ACS_GUI out"=w7496:refnum<class "S4GUI.lvclass">)  [unwired: 7 in]
        n3073 = call "Read WPSEL.vi"("error in (no error)"=w7504, "Instrument in"=w7505) -> ("error out"=w7501:errorcluster, "Opt_Selector.lvclass"=w7503:refnum<class "Opt_Selector.lvclass">, "Instrument out"=w7499:refnum<class "Instrument.lvclass">)  [unwired: 7 in]
        n3074 = call "Write target.vi"("error in (no error)"=w7501, "target"=w7502, "Optics in"=w7503) -> ("error out"=w7498:errorcluster, "Optics out"=w7500:refnum<class "Opt_Selector.lvclass">)  [unwired: 7 in]
        n3075 = call "Write WPSEL.vi"("error in (no error)"=w7498, "Opt_Selector.lvclass"=w7500, "Instrument in"=w7499) -> ("error out"=w7495:errorcluster, "Instrument out"=w7497:refnum<class "Instrument.lvclass">)  [unwired: 7 in]
        n3076 = call "Write Instrument.lvclass.vi"("error in (no error)"=w7495, "Instrument.lvclass"=w7497, "S4ACS_GUI in"=w7496) -> ("error out"=w7494:errorcluster, "S4ACS_GUI out"=w7493:refnum<class "S4GUI.lvclass">)  [unwired: 7 in]
      }
      event "WPSEL_set": Value Change {
        n3077 = event-data() -> ()  [unwired: 1 in, 4 out]
        n3078 = call "Read Instrument.lvclass.vi"("error in (no error)"=w7526, "S4ACS_GUI in"=w7527) -> ("error out"=w7524:errorcluster, "Instrument.lvclass"=w7525:refnum<class "Instrument.lvclass">, "S4ACS_GUI out"=w7512:refnum<class "S4GUI.lvclass">)  [unwired: 7 in]
        n3079 = call "Read WPSEL.vi"("error in (no error)"=w7524, "Instrument in"=w7525) -> ("error out"=w7521:errorcluster, "Opt_Selector.lvclass"=w7523:refnum<class "Opt_Selector.lvclass">, "Instrument out"=w7515:refnum<class "Instrument.lvclass">)  [unwired: 7 in]
        n3080 = call-dynamic "Read State Machine.vi"("error in (no error)"=w7521, "Device in"=w7523) -> ("error out"=w7520:errorcluster, "State Machine.lvclass"=w7509:refnum<class "State Machine.lvclass">, "Device out"=w7517:refnum<class "Opt_Selector.lvclass">)  [unwired: 7 in]
        n3081 = call "Next State.vi"("error in (no error)"=w7520, "New_State"=1, "State Machine in"=w7509) -> ("error out"=w7519:errorcluster, "State Machine out"=w7518:refnum<class "State Machine.lvclass">)  [unwired: 7 in]
        n3082 = call-dynamic "Write State Machine.vi"("error in (no error)"=w7519, "State Machine.lvclass"=w7518, "Device in"=w7517) -> ("error out"=w7514:errorcluster, "Device out"=w7516:refnum<class "Opt_Selector.lvclass">)  [unwired: 7 in]
        n3083 = call "Write WPSEL.vi"("error in (no error)"=w7514, "Opt_Selector.lvclass"=w7516, "Instrument in"=w7515) -> ("error out"=w7511:errorcluster, "Instrument out"=w7513:refnum<class "Instrument.lvclass">)  [unwired: 7 in]
        n3084 = call "Write Instrument.lvclass.vi"("error in (no error)"=w7511, "Instrument.lvclass"=w7513, "S4ACS_GUI in"=w7512) -> ("error out"=w7510:errorcluster, "S4ACS_GUI out"=w7508:refnum<class "S4GUI.lvclass">)  [unwired: 7 in]
      }
      event "Set Waveplate": Value Change {
        # "Garantir que, quando em POLARIMETRIA, pelo menos WP1 esteja selecionado."
        # "aqui também"
        # "OV20230426: Montagem do CALW\nestá com POL e DEPOL invertidos"
        n3085 = event-data() -> ()  [unwired: 1 in, 4 out]
        n3086 = local read "Calibrator Selector"() -> (w7599:u16)
        n3087 = call "Read Instrument.lvclass.vi"("error in (no error)"=w7597, "S4ACS_GUI in"=w7596) -> ("error out"=w7616:errorcluster, "Instrument.lvclass"=w7617:refnum<class "Instrument.lvclass">, "S4ACS_GUI out"=w7614:refnum<class "S4GUI.lvclass">)  [unwired: 7 in]
        n3088 = property on="Calibrator Selector" class="Ring (strict)"() -> ("RingText.Text"=w7598:string)  [unwired: 2 in, 2 out]
        n3089 = property on="Lambda Selector" class="Ring (strict)"() -> ("RingText.Text"=w7619:string)  [unwired: 2 in, 2 out]
        n3090 = Build Array(0.0 ("element"), 288.0 ("element"), 144.0 ("element"), 216.0 ("element"), 72.0 ("element")) -> (w7610:dbl[])
        n3091 = local read "Lambda Selector"() -> (w7618:u16)
        n3092 = call "Read CALW.vi"("error in (no error)"=w7616, "Instrument in"=w7617) -> ("error out"=w7608:errorcluster, "Opt_Selector.lvclass"=w7607:refnum<class "Opt_Selector.lvclass">, "Instrument out"=w7615:refnum<class "Instrument.lvclass">)  [unwired: 7 in]
        n3093 = Index Array(array=w7610, index=w7599) -> (element=w7609:dbl)
        n3094 = Build Array(80.0 ("element"), 0.0 ("element"), 160.0 ("element")) -> (w7646:dbl[])
        n3095 = call "Write target.vi"("error in (no error)"=w7608, "target"=w7609, "Optics in"=w7607) -> ("error out"=w7605:errorcluster, "Optics out"=w7606:refnum<class "Opt_Selector.lvclass">)  [unwired: 7 in]
        n3096 = case shown="\"DEPOLARIZER\"" w7598 {
          tunnel: ["OFF" w7875 "PINHOLE" "SHUTTER" w7880] -> w7602
          frame "OFF", Default {
          }
          frame "POLARIZER" {
            n3097 = disable-structure shown="Enabled" {
              disable-tunnel: ["POLARIZER" "DEPOLARIZER"] -> w7875
              frame Disabled {
              }
              frame Enabled {
                # "OV20230426: Montagem do CALW\nestá com POL e DEPOL invertidos"
              }
            }
          }
          frame "PINHOLE" {
          }
          frame "SHUTTER" {
          }
          frame "DEPOLARIZER" {
            n3098 = disable-structure shown="Enabled" {
              disable-tunnel: ["POLARIZER" "DEPOLARIZER"] -> w7880
              frame Enabled {
                # "OV20230426: Montagem do CALW\nestá com POL e DEPOL invertidos"
              }
              frame Disabled {
              }
            }
          }
        }
        n3099 = Index Array(array=w7646, index=w7618) -> (element=w7645:dbl)
        n3100 = case shown="\"OFF\", Default" w7619 {
          tunnel: [w7883 "ON" "ON"] -> w7637
          tunnel: [0.0 ("element") 30.0 ("element") 30.0 ("element")] -> w7636
          tunnel: [w7883 "L/2" "L/4"] -> w7629
          frame "OFF", Default {
            w7883 = "OFF"
          }
          frame "Lambda/2" {
          }
          frame "Lambda/4" {
          }
        }
        n3101 = call "Write target name.vi"("error in (no error)"=w7605, "target name"=w7602, "Optics in"=w7606) -> ("error out"=w7604:errorcluster, "Optics out"=w7603:refnum<class "Opt_Selector.lvclass">)  [unwired: 7 in]
        n3102 = call "Write CALW.vi"("error in (no error)"=w7604, "Opt_Selector.lvclass"=w7603, "Instrument in"=w7615) -> ("error out"=w7600:errorcluster, "Instrument out"=w7601:refnum<class "Instrument.lvclass">)  [unwired: 7 in]
        n3103 = call "Write Instrument.lvclass.vi"("error in (no error)"=w7600, "Instrument.lvclass"=w7601, "S4ACS_GUI in"=w7614) -> ("error out"=w7594:errorcluster, "S4ACS_GUI out"=w7595:refnum<class "S4GUI.lvclass">)  [unwired: 7 in]
        n3104 = call "Read Instrument.lvclass.vi"("error in (no error)"=w7594, "S4ACS_GUI in"=w7595) -> ("error out"=w7650:errorcluster, "Instrument.lvclass"=w7628:refnum<class "Instrument.lvclass">, "S4ACS_GUI out"=w7626:refnum<class "S4GUI.lvclass">)  [unwired: 7 in]
        n3105 = call "Read WPSEL.vi"("error in (no error)"=w7650, "Instrument in"=w7628) -> ("error out"=w7635:errorcluster, "Opt_Selector.lvclass"=w7634:refnum<class "Opt_Selector.lvclass">, "Instrument out"=w7627:refnum<class "Instrument.lvclass">)  [unwired: 7 in]
        n3106 = call "Write target.vi"("error in (no error)"=w7635, "target"=w7645, "Optics in"=w7634) -> ("error out"=w7632:errorcluster, "Optics out"=w7633:refnum<class "Opt_Selector.lvclass">)  [unwired: 7 in]
        n3107 = call "Write target name.vi"("error in (no error)"=w7632, "target name"=w7629, "Optics in"=w7633) -> ("error out"=w7631:errorcluster, "Optics out"=w7630:refnum<class "Opt_Selector.lvclass">)  [unwired: 7 in]
        n3108 = call "Write WPSEL.vi"("error in (no error)"=w7631, "Opt_Selector.lvclass"=w7630, "Instrument in"=w7627) -> ("error out"=w7623:errorcluster, "Instrument out"=w7622:refnum<class "Instrument.lvclass">)  [unwired: 7 in]
        n3109 = call "Read ASEL.vi"("error in (no error)"=w7623, "Instrument in"=w7622) -> ("error out"=w7642:errorcluster, "Opt_Selector.lvclass"=w7640:refnum<class "Opt_Selector.lvclass">, "Instrument out"=w7625:refnum<class "Instrument.lvclass">)  [unwired: 7 in]
        n3110 = call "Write target name.vi"("error in (no error)"=w7642, "target name"=w7637, "Optics in"=w7640) -> ("error out"=w7643:errorcluster, "Optics out"=w7639:refnum<class "Opt_Selector.lvclass">)  [unwired: 7 in]
        n3111 = call "Write target.vi"("error in (no error)"=w7643, "target"=w7636, "Optics in"=w7639) -> ("error out"=w7644:errorcluster, "Optics out"=w7638:refnum<class "Opt_Selector.lvclass">)  [unwired: 7 in]
        n3112 = call "Write ASEL.vi"("error in (no error)"=w7644, "Opt_Selector.lvclass"=w7638, "Instrument in"=w7625) -> ("error out"=w7641:errorcluster, "Instrument out"=w7624:refnum<class "Instrument.lvclass">)  [unwired: 7 in]
        n3113 = call "Write Instrument.lvclass.vi"("error in (no error)"=w7641, "Instrument.lvclass"=w7624, "S4ACS_GUI in"=w7626) -> ("error out"=w7620:errorcluster, "S4ACS_GUI out"=w7621:refnum<class "S4GUI.lvclass">)  [unwired: 7 in]
        n3114 = call "Read Instrument.lvclass.vi"("error in (no error)"=w7620, "S4ACS_GUI in"=w7621) -> ("error out"=w7691:errorcluster, "Instrument.lvclass"=w7692:refnum<class "Instrument.lvclass">, "S4ACS_GUI out"=w7532:refnum<class "S4GUI.lvclass">)  [unwired: 7 in]
        n3115 = call "Read WPSEL.vi"("error in (no error)"=w7691, "Instrument in"=w7692) -> ("error out"=w7688:errorcluster, "Opt_Selector.lvclass"=w7690:refnum<class "Opt_Selector.lvclass">, "Instrument out"=w7682:refnum<class "Instrument.lvclass">)  [unwired: 7 in]
        n3116 = call-dynamic "Read State Machine.vi"("error in (no error)"=w7688, "Device in"=w7690) -> ("error out"=w7687:errorcluster, "State Machine.lvclass"=w7680:refnum<class "State Machine.lvclass">, "Device out"=w7684:refnum<class "Opt_Selector.lvclass">)  [unwired: 7 in]
        n3117 = call "Next State.vi"("error in (no error)"=w7687, "New_State"=1, "State Machine in"=w7680) -> ("error out"=w7686:errorcluster, "State Machine out"=w7685:refnum<class "State Machine.lvclass">)  [unwired: 7 in]
        n3118 = call-dynamic "Write State Machine.vi"("error in (no error)"=w7686, "State Machine.lvclass"=w7685, "Device in"=w7684) -> ("error out"=w7681:errorcluster, "Device out"=w7683:refnum<class "Opt_Selector.lvclass">)  [unwired: 7 in]
        n3119 = call "Write WPSEL.vi"("error in (no error)"=w7681, "Opt_Selector.lvclass"=w7683, "Instrument in"=w7682) -> ("error out"=w7672:errorcluster, "Instrument out"=w7671:refnum<class "Instrument.lvclass">)  [unwired: 7 in]
        n3120 = call "Read ASEL.vi"("error in (no error)"=w7672, "Instrument in"=w7671) -> ("error out"=w7678:errorcluster, "Opt_Selector.lvclass"=w7669:refnum<class "Opt_Selector.lvclass">, "Instrument out"=w7670:refnum<class "Instrument.lvclass">)  [unwired: 7 in]
        n3121 = call-dynamic "Read State Machine.vi"("error in (no error)"=w7678, "Device in"=w7669) -> ("error out"=w7677:errorcluster, "State Machine.lvclass"=w7673:refnum<class "State Machine.lvclass">, "Device out"=w7668:refnum<class "Opt_Selector.lvclass">)  [unwired: 7 in]
        n3122 = call "Next State.vi"("error in (no error)"=w7677, "New_State"=1, "State Machine in"=w7673) -> ("error out"=w7676:errorcluster, "State Machine out"=w7675:refnum<class "State Machine.lvclass">)  [unwired: 7 in]
        n3123 = call-dynamic "Write State Machine.vi"("error in (no error)"=w7676, "State Machine.lvclass"=w7675, "Device in"=w7668) -> ("error out"=w7674:errorcluster, "Device out"=w7667:refnum<class "Opt_Selector.lvclass">)  [unwired: 7 in]
        n3124 = call "Write ASEL.vi"("error in (no error)"=w7674, "Opt_Selector.lvclass"=w7667, "Instrument in"=w7670) -> ("error out"=w7654:errorcluster, "Instrument out"=w7656:refnum<class "Instrument.lvclass">)  [unwired: 7 in]
        n3125 = call "Read CALW.vi"("error in (no error)"=w7654, "Instrument in"=w7656) -> ("error out"=w7664:errorcluster, "Opt_Selector.lvclass"=w7666:refnum<class "Opt_Selector.lvclass">, "Instrument out"=w7655:refnum<class "Instrument.lvclass">)  [unwired: 7 in]
        n3126 = call-dynamic "Read State Machine.vi"("error in (no error)"=w7664, "Device in"=w7666) -> ("error out"=w7663:errorcluster, "State Machine.lvclass"=w7657:refnum<class "State Machine.lvclass">, "Device out"=w7660:refnum<class "Opt_Selector.lvclass">)  [unwired: 7 in]
        n3127 = call "Next State.vi"("error in (no error)"=w7663, "New_State"=1, "State Machine in"=w7657) -> ("error out"=w7662:errorcluster, "State Machine out"=w7661:refnum<class "State Machine.lvclass">)  [unwired: 7 in]
        n3128 = property on="Lambda Selector" class="Ring (strict)"() -> ("RingText.Text"=w7653:string)  [unwired: 2 in, 2 out]
        n3129 = call-dynamic "Write State Machine.vi"("error in (no error)"=w7662, "State Machine.lvclass"=w7661, "Device in"=w7660) -> ("error out"=w7658:errorcluster, "Device out"=w7659:refnum<class "Opt_Selector.lvclass">)  [unwired: 7 in]
        n3130 = call "Write CALW.vi"("error in (no error)"=w7658, "Opt_Selector.lvclass"=w7659, "Instrument in"=w7655) -> ("error out"=w7531:errorcluster, "Instrument out"=w7652:refnum<class "Instrument.lvclass">)  [unwired: 7 in]
        n3131 = call-dynamic "Read mode EXPOSE.vi"("error in (no error)"=w7531, "S4GUI in"=w7532) -> ("error out"=w7530:errorcluster, "mode EXPOSE"=w7528:bool, "S4GUI out"=w7529:refnum<class "S4GUI.lvclass">)  [unwired: 7 in]
        n3132 = call-dynamic "Read sync.vi"("error in (no error)"=w7530, "S4ACS_GUI in"=w7529) -> ("error out"=w7551:errorcluster, "sync"=w7550:bool, "S4ACS_GUI out"=w7552:refnum<class "S4GUI.lvclass">)  [unwired: 7 in]
        n3133 = case shown="Default" w7653 {
          selector: w7653 -> [w7900 _]
          tunnel: w7652 -> [w7904 w7922]
          tunnel: [w7903 w7922] -> w7651
          tunnel: [w7896 w7921] -> w7568
          tunnel: w7551 -> [w7902 w7921]
          tunnel: [w7893 w7917] -> w7563
          tunnel: w7550 -> [w7892 _]
          tunnel: w7528 -> [w7891 w7920]
          frame "OFF" {
            w7894 = u16 0 items=["OFF", "POLARIZER", "PINHOLE", "SHUTTER", "DEPOLARIZER"] ("Calibrator Selector 2")
            n3134 = call "Read CALW.vi"("error in (no error)"=w7902, "Instrument in"=w7904) -> ("error out"=w7907:errorcluster, "Opt_Selector.lvclass"=w7909:refnum<class "Opt_Selector.lvclass">, "Instrument out"=w7908:refnum<class "Instrument.lvclass">)  [unwired: 7 in]
            n3135 = call "Write target.vi"("error in (no error)"=w7907, "target"=0.0, "Optics in"=w7909) -> ("error out"=w7906:errorcluster, "Optics out"=w7910:refnum<class "Opt_Selector.lvclass">)  [unwired: 7 in]
            n3136 = call "Write target name.vi"("error in (no error)"=w7906, "target name"=w7900, "Optics in"=w7910) -> ("error out"=w7905:errorcluster, "Optics out"=w7911:refnum<class "Opt_Selector.lvclass">)  [unwired: 7 in]
            n3137 = call "Write CALW.vi"("error in (no error)"=w7905, "Opt_Selector.lvclass"=w7911, "Instrument in"=w7908) -> ("error out"=w7895:errorcluster, "Instrument out"=w7903:refnum<class "Instrument.lvclass">)  [unwired: 7 in]
            n3138 = property on="Calibrator Selector" class="Ring (strict)"(error in=w7895, "Value"=w7894, "DisabledEnum"=T7."Disabled and Grayed Out" ("Disabled")) -> (error out=w7897:errorcluster)  [unwired: 1 in, 1 out]
            n3139 = property on="Calibrator Selector" class="Ring (strict)"(error in=w7897, "RingText.Text"="OFF" ("Ring Text.Text")) -> (error out=w7896:errorcluster)  [unwired: 1 in, 1 out]
            n3140 = case shown="True" w7892 {
              tunnel: [u8 0 ("SHUTTER_MODE") w7914] -> w7893
              tunnel: w7891 -> [_ w7913]
              frame False {
                # "Fotom. & Async"
                # "Internal"
              }
              frame True {
                # "Ext. Start"
                # "Internal"
                # "Fotom. Sync. SEM exp mode"
                # "Fotom. Sync. COM exp mode"
                n3141 = Select(t=u8 0, s=w7913, f=u8 6 ("SHUTTER_MODE")) -> (s? t:f=w7914:u8)
              }
            }
          }
          frame Default {
            # "Polar. COM exp mode"
            # "Internal"
            # "Polar. SEM exp mode"
            # "Ext. Start"
            n3142 = Select(t=u8 0, s=w7920, f=u8 6 ("SHUTTER_MODE")) -> (s? t:f=w7917:u8)
          }
        }
        n3143 = call "Write Instrument.lvclass.vi"("error in (no error)"=w7568, "Instrument.lvclass"=w7651, "S4ACS_GUI in"=w7552) -> ("error out"=w7567:errorcluster, "S4ACS_GUI out"=w7556:refnum<class "S4GUI.lvclass">)  [unwired: 7 in]
        n3144 = call-dynamic "Read AcquisitionC.vi"("error in (no error)"=w7567, "S4ACS_GUI in"=w7556) -> ("error out"=w7578:errorcluster, "Acquisition.lvclass"=w7577:refnum<class "Acquisition.lvclass">)  [unwired: 7 in, 1 out]
